vi "Calculadora Altitud.vi"() -> ()   [LabVIEW 2019]
panel:
  out "?":enum32{"Page 1", "Page 2", "Page 3"}(tab)
  in  "?":bool
  in  "?":bool
  in  "?":dbl
  in  "m":string(combo)
  in  "?":bool
  in  "?":bool
  out "?":dbl
  out "?":dbl(slide) scale=0.0..20000.0
  in  "?":bool
  out "Densidad 1":dbl
  out "Presion":dbl
  out "Temperatura":dbl
  # "Bienvenido a la calculadora de \ndensidad, presión y temperatura del aire frente a la Altitud"
  # "Kevin Castañeda"
  # "Hecho por:"
  # "Ingresa la altitud de la aeronave y la unidad de medida"
  # "Altitud en metros"
  # "°K"
  # "Pa"
  # "Estratosfera"
  # "/"
  # "Kg"
  # "3"
  # "m"
  # "Tropopausa"
  # "m"
  # "Troposfera"
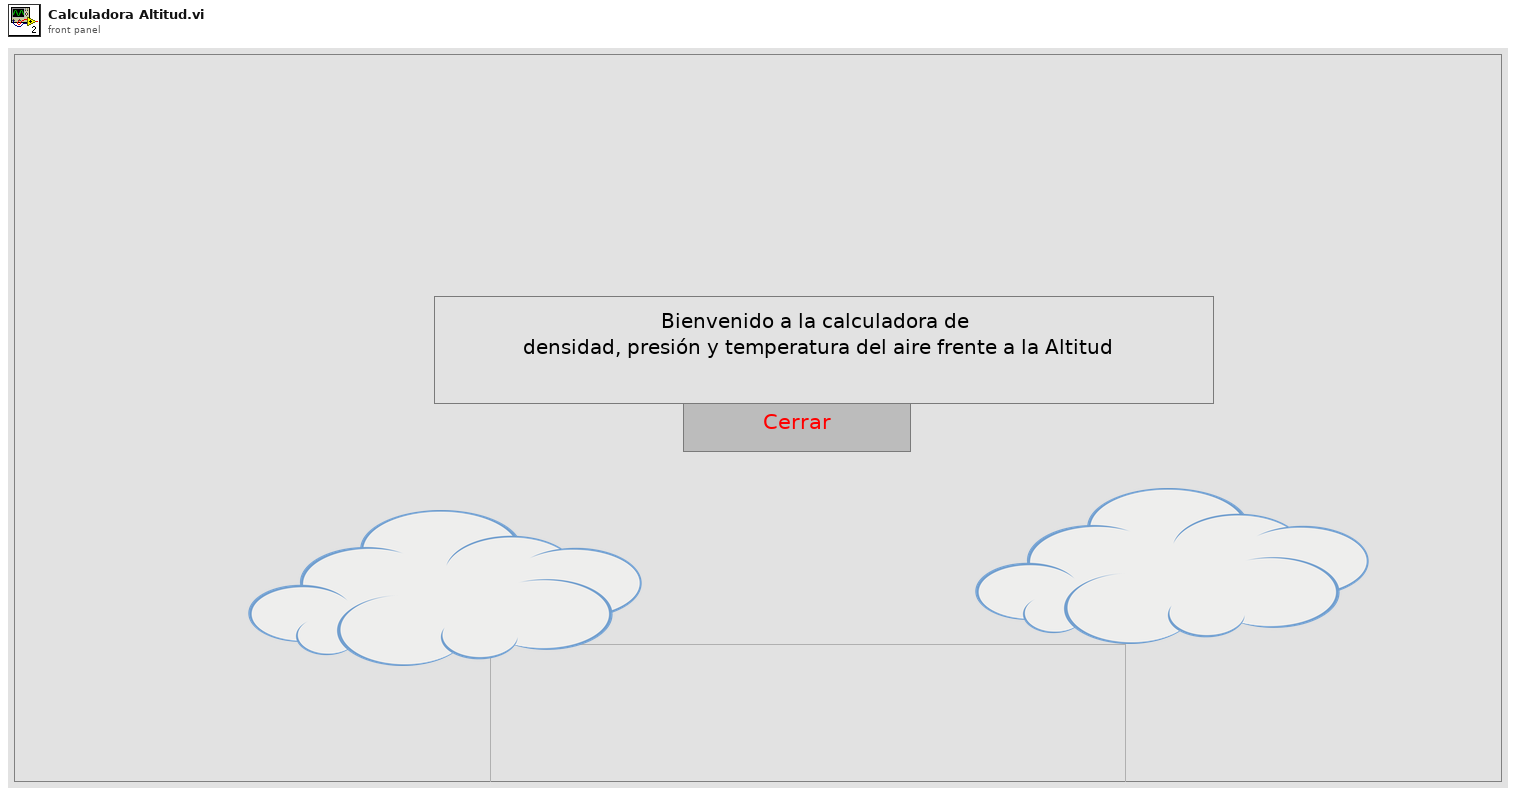
[diagram p1: front panel]
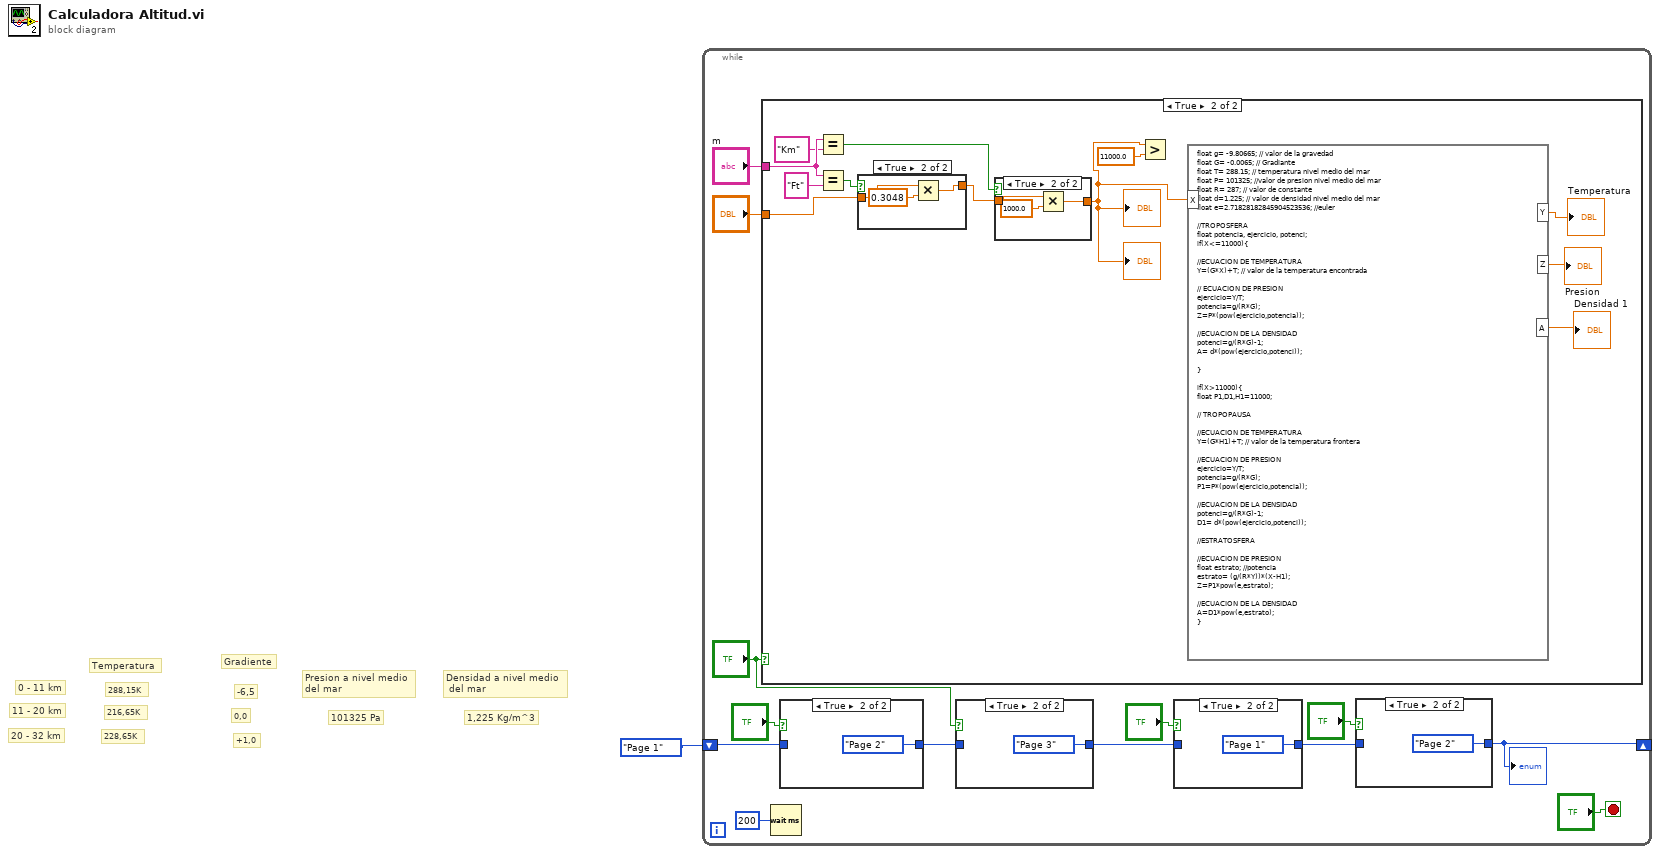
[diagram p0: block diagram]
diagram:
  # "1,225 Kg/m^3"
  # "Densidad a nivel medio\n del mar"
  # "101325 Pa"
  # "Presion a nivel medio\ndel mar"
  # "+1,0"
  # "0,0"
  # "-6,5"
  # "Gradiente"
  # "228,65K"
  # "20 - 32 km"
  # "216,65K"
  # "11 - 20 km"
  # "288,15K"
  # "0 - 11 km"
  # "Temperatura"
  n1 = while {
    shift-right: [w4] -> _
    shift-left: enum32{"Page 1", "Page 2", "Page 3"}."Page 1" -> [w10]
    stop <- "?" stop-if-true
    n2 = case shown="True" "?" {
      tunnel: "?" -> [_ w32]
      tunnel: "m" -> [_ w31]
      frame False {
      }
      frame True {
        n3 = Equal?(x=w31, y="Km") -> (x = y?=w29:bool)
        n4 = Equal?(x=w31, y="Ft") -> (x = y?=w33:bool)
        n5 = case shown="True" w33 {
          tunnel: w32 -> [w39 w42]
          tunnel: [w39 w40] -> w28
          frame False {
          }
          frame True {
            n6 = Multiply(x=w42, y=0.3048) -> (x*y=w40:dbl)
          }
        }
        n7 = case shown="True" w29 {
          tunnel: w28 -> [w35 w38]
          tunnel: [w35 w36] -> w26
          frame False {
          }
          frame True {
            n8 = Multiply(x=w38, y=1000.0) -> (x*y=w36:dbl)
          }
        }
        "?" <- w26
        "?" <- w26
        n9 = Greater?(x=w26, y=11000.0) -> ()  [unwired: 1 out]
        n10 = formula code="float g= -9.80665; // valor de la gravedad\nfloat G= -0.0065; // Gradiante \nfloat T= 288.15; // temperatura nivel medio del mar\nfloat P= 101325; //valor de presion nivel medio del mar\nfloat R= 287; // valor de constante \nfloat d=1.225; // valor de densidad nivel medio del mar\nfloat e=2.71828182845904523536; //euler\n\n//TROPOSFERA\nfloat potencia, ejercicio, potenci;\nif(X<=11000){\n\n//ECUACION DE TEMPERATURA\nY=(G*X)+T; // valor de la temperatura encontrada\n\n// ECUACION DE PRESION\nejercicio=Y/T;\npotencia=g/(R*G);\nZ=P*(pow(ejercicio,potencia));\n\n//ECUACION DE LA DENSIDAD\npotenci=g/(R*G)-1;\nA= d*(pow(ejercicio,potenci));\n\n}\n\nif(X>11000){ \nfloat P1,D1,H1=11000;\n\n// TROPOPAUSA\n\n//ECUACION DE TEMPERATURA\nY=(G*H1)+T; // valor de la temperatura frontera\n\n//ECUACION DE PRESION\nejercicio=Y/T;\npotencia=g/(R*G);\nP1=P*(pow(ejercicio,potencia));\n\n//ECUACION DE LA DENSIDAD\npotenci=g/(R*G)-1;\nD1= d*(pow(ejercicio,potenci));\n\n//ESTRATOSFERA\n\n//ECUACION DE PRESION\nfloat estrato; //potencia\nestrato= (g/(R*Y))*(X-H1);\nZ=P1*pow(e,estrato);\n\n//ECUACION DE LA DENSIDAD\nA=D1*pow(e,estrato);\n}"("X"=w26) -> ("Y"=→"Temperatura":dbl, "Z"=→"Presion":dbl, "A"=→"Densidad 1":dbl)
      }
    }
    n11 = Wait (ms)(milliseconds to wait=u32 200) -> ()  [unwired: 1 out]
    n12 = case shown="True" "?" {
      tunnel: [w21 enum32{"Page 1", "Page 2", "Page 3"}."Page 2"] -> w9
      tunnel: w10 -> [w21 _]
      frame False {
      }
      frame True {
      }
    }
    n13 = case shown="True" "?" {
      tunnel: [w19 enum32{"Page 1", "Page 2", "Page 3"}."Page 3"] -> w7
      tunnel: w9 -> [w19 _]
      frame False {
      }
      frame True {
      }
    }
    n14 = case shown="True" "?" {
      tunnel: [w17 enum32{"Page 1", "Page 2", "Page 3"}."Page 1"] -> w3
      tunnel: w7 -> [w17 _]
      frame False {
      }
      frame True {
      }
    }
    n15 = case shown="True" "?" {
      tunnel: [w15 enum32{"Page 1", "Page 2", "Page 3"}."Page 2"] -> w4
      tunnel: w3 -> [w15 _]
      frame False {
      }
      frame True {
      }
    }
    "?" <- w4
  }
